vi "tracking+matching_gige_mit_5_pattern.vi"() -> ()   [LabVIEW 2014]
uses:
  <vilib>/userdefined/High Color/IMAQdx.ctl
  <vilib>/vision/Avi1.llb/AviRefnum.ctl
  <vilib>/vision/driver/NI_Vision_Acquisition_Software.lvlib
  <vilib>/vision/NI_Vision_Development_Module.lvlib
  <resource>/objmgr/imaqdx.rc
panel:
  in  "Max Data Size":u32=10000
  out "Selected Path":path
  in  "Frames Per Second":u32=20
  in  "BayerPattern":u32(ring)=5 items=["None", "GB", "GR", "BG", "RG", "Use Hardware Value"]
  out "ValueString":string
  out "ValueBool":bool
  out "IPAddress":string
  in  "Aufnahme Starten":bool
  in  "pattern5":bool
  in  "Pattern5 Farbe":u32(colorbox)=16711680
  in  "y":i32
  in  "x":i32
  out "Pattern 5":T1(plugin-control)
  in  "Template File Path (Pattern Matching 5)":path=path "C:/Users/Kroll/Desktop/Test_04012016/Pattern/pattern_1412.png"
  in  "pattern4":bool
  in  "Pattern4 Farbe":u32(colorbox)=16711680
  in  "y":i32
  in  "x":i32
  out "Pattern 4":T1(plugin-control)
  in  "Template File Path (Pattern Matching 4)":path=path "C:/Users/Kroll/Desktop/Test_04012016/Pattern/pattern_1412.png"
  in  "pattern3":bool
  in  "Pattern3 Farbe":u32(colorbox)=16711680
  in  "y":i32
  in  "x":i32
  out "Pattern 3":T1(plugin-control)
  in  "Template File Path (Pattern Matching 3)":path=path "C:/Users/Kroll/Desktop/Test_04012016/Pattern/pattern_1412.png"
  in  "pattern2":bool
  in  "Pattern2 Farbe":u32(colorbox)=16711680
  in  "x":i32
  in  "y":i32
  out "Pattern 2":T1(plugin-control)
  in  "Template File Path (Pattern Matching 2)":path=path "C:/Users/Kroll/Desktop/Test_04012016/Pattern/pattern_1412.png"
  out "date/time string":string
  in  "file path (dialog if empty)":path=path "I:/123.txt"
  in  "Länge der Spur":i32=50
  out "Pattern1":T1(plugin-control)
  in  "Template File Path (Pattern Matching 1)":path=path "C:/Users/Kroll/Desktop/Test_04012016/Pattern/pattern_1412.png"
  out "Image 2":T1(plugin-control)
  in  "Programm anhalten":bool
  in  "Parameters Pattern":T2={"Number of Matches Requested"=1, "Minimum Match Score"=800.0, "Angle Ranges"=[{"Start Angle"=-180.0, "End Angle"=180.0}, {"Start Angle"=0.0, "End Angle"=360.0}]}
  in  "Mittelpunktgröße":sgl
  in  "millisecond multiple":u32
  out "Processed Frames/s":dbl
  in  "Länge des Pfeils":sgl=80.0
  out "Acquired Frames/s":dbl
  in  "pattern1":bool
  in  "Pattern1 Farbe":u32(colorbox)=16711680
  in  "x":i32
  in  "y":i32
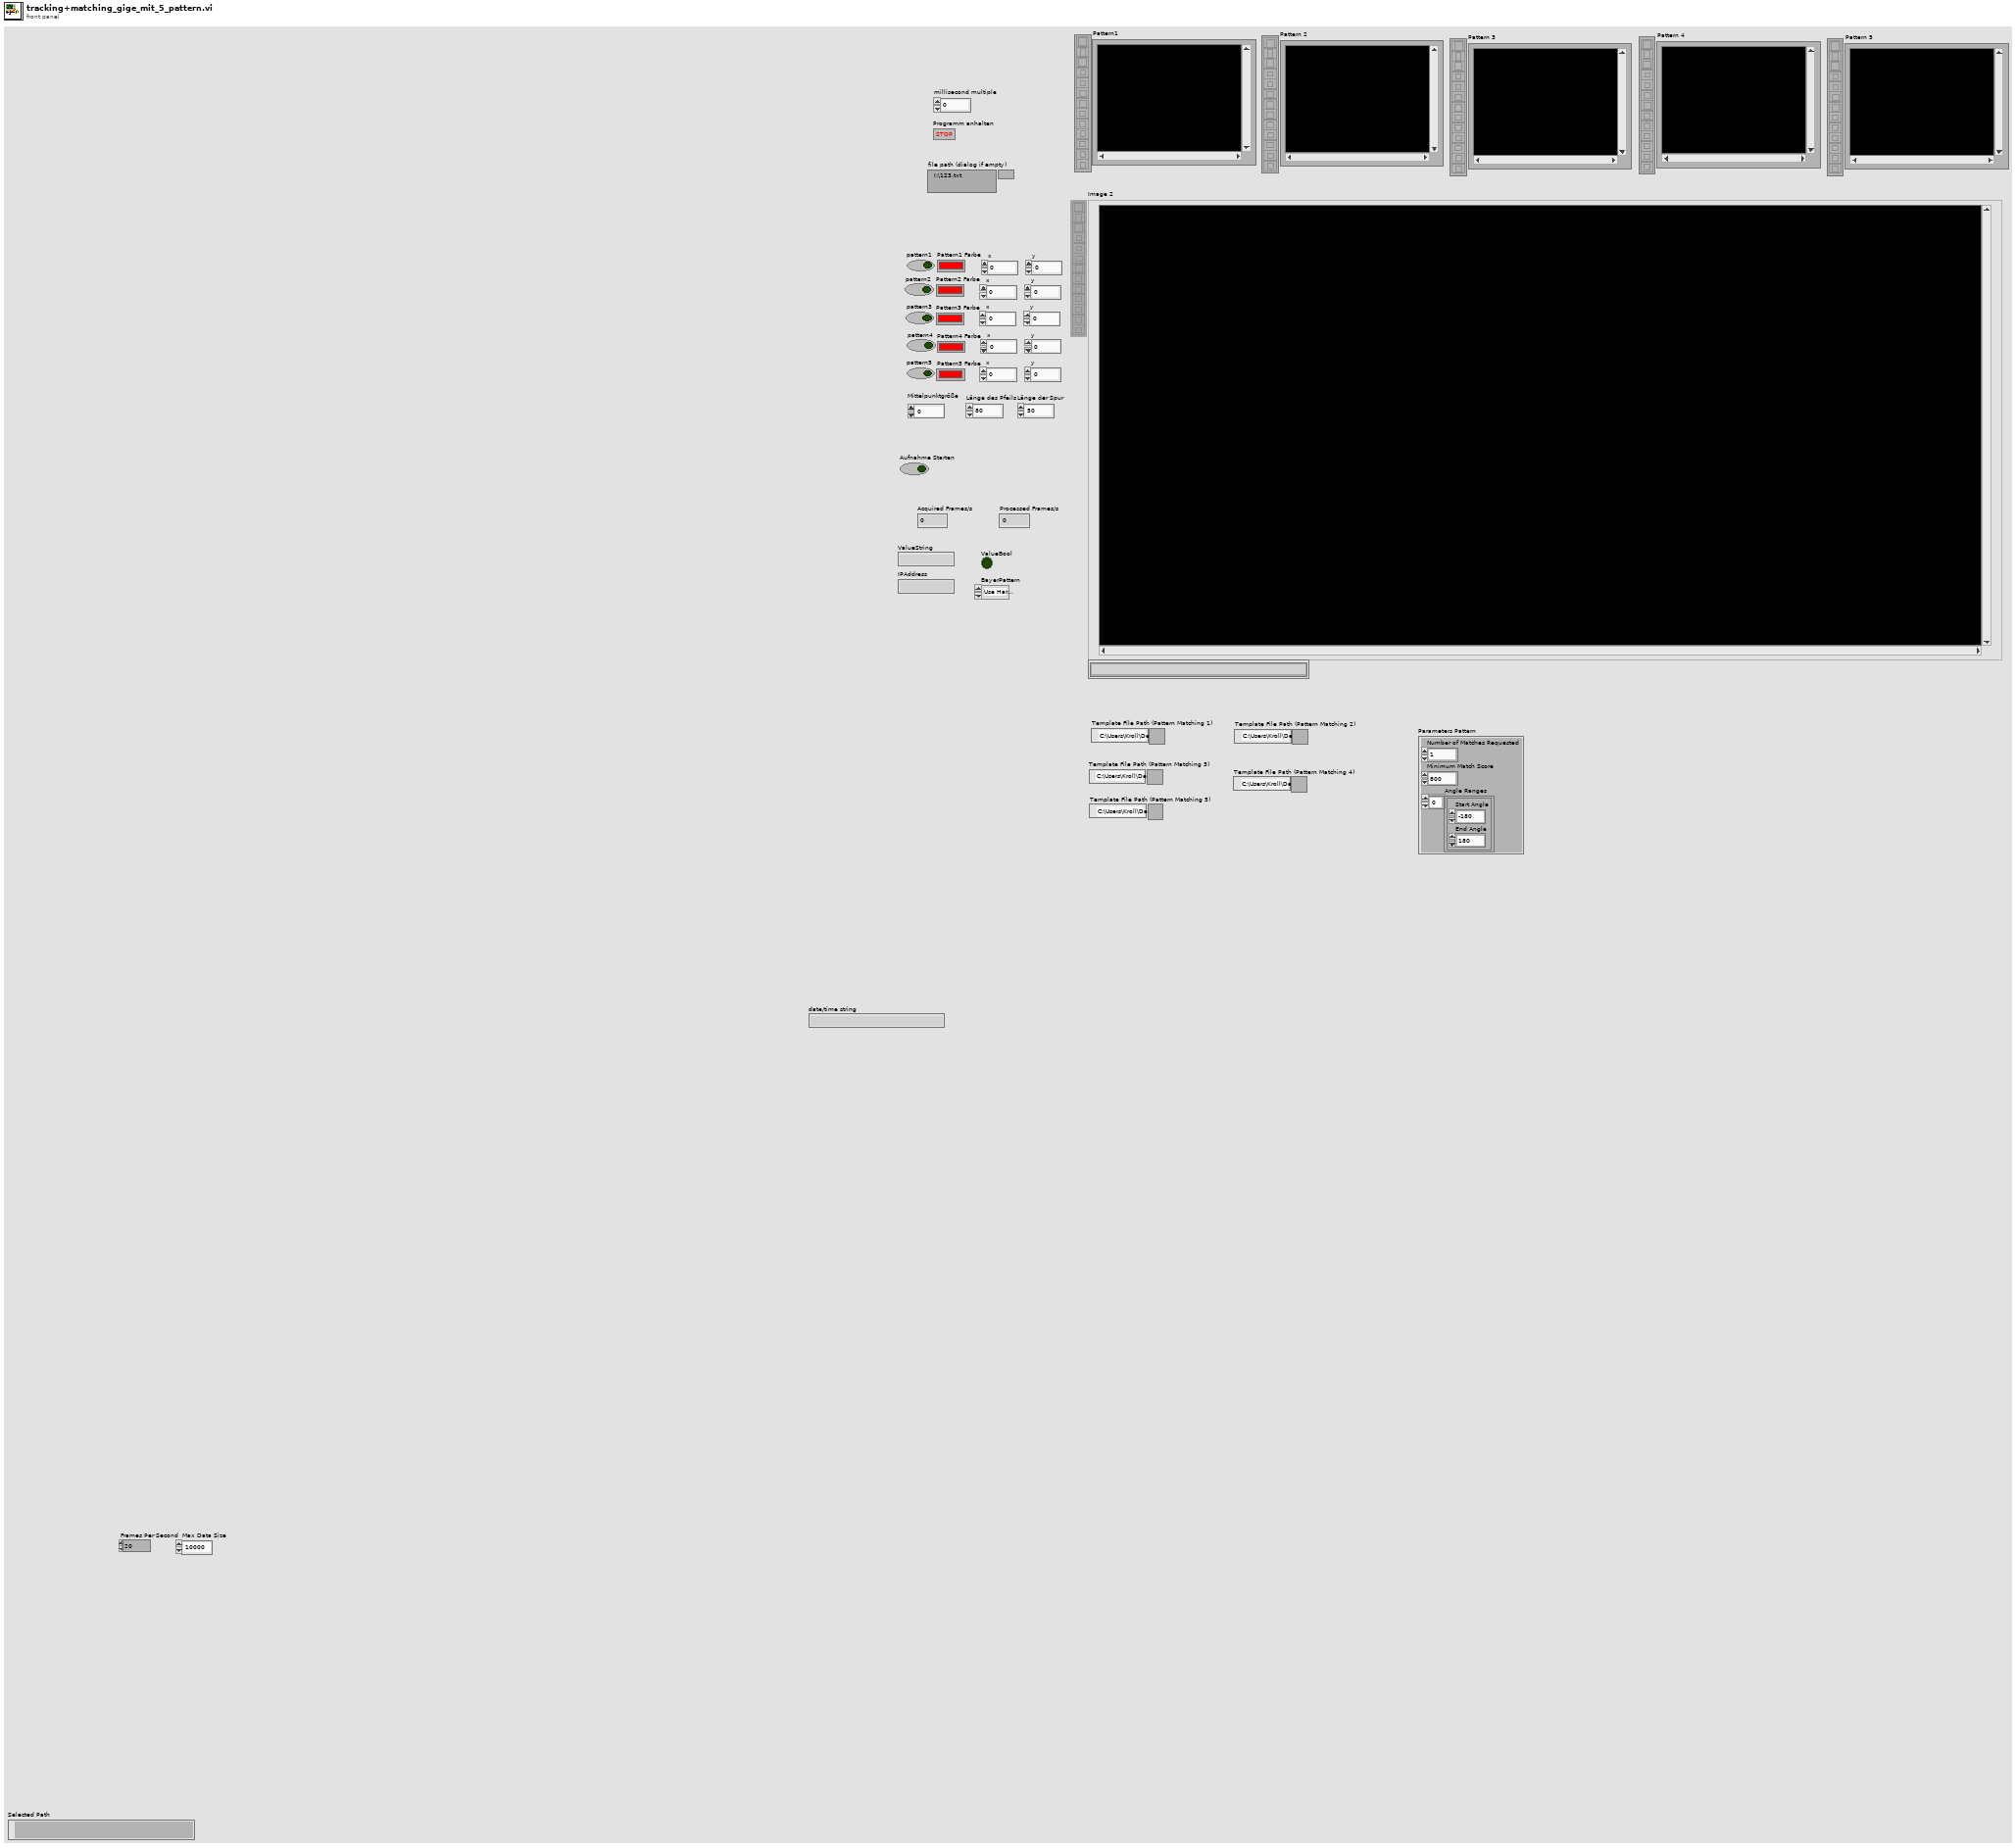
[diagram p1: front panel]
types:
  T1 = typedef "IMAQ Image.ctl" = refnum<image>
  T2 = cluster{"Number of Matches Requested":i32, "Minimum Match Score":sgl, "Angle Ranges":cluster{"Start Angle":sgl, "End Angle":sgl}[]}
  T3 = typedef "IMAQdx.ctl" = refnum<k21>
  T4 = cluster{"Number of Histogram Bins":i32, "Blending Parameter (%)":dbl, "Maximum Iterations":i32}
  T5 = typedef "Image Type" = u32
  T6 = enum16{"open", "replace", "create", "open or create", "replace or create", "replace or create with confirmation"}
  T7 = typedef "AviRefnum.ctl" = refnum<k1>
  T8 = enum32{"existing file", "new file", "new or existing file", "existing dir", "new dir", "new or existing dir", "existing file (use LLBs)", "new file (use LLBs)", "new or existing file (use LLBs)", "new or existing file or directory (use LLBs)"}
  T9 = typedef "IMAQ Object Tracking Session.ctl" = refnum<k20>
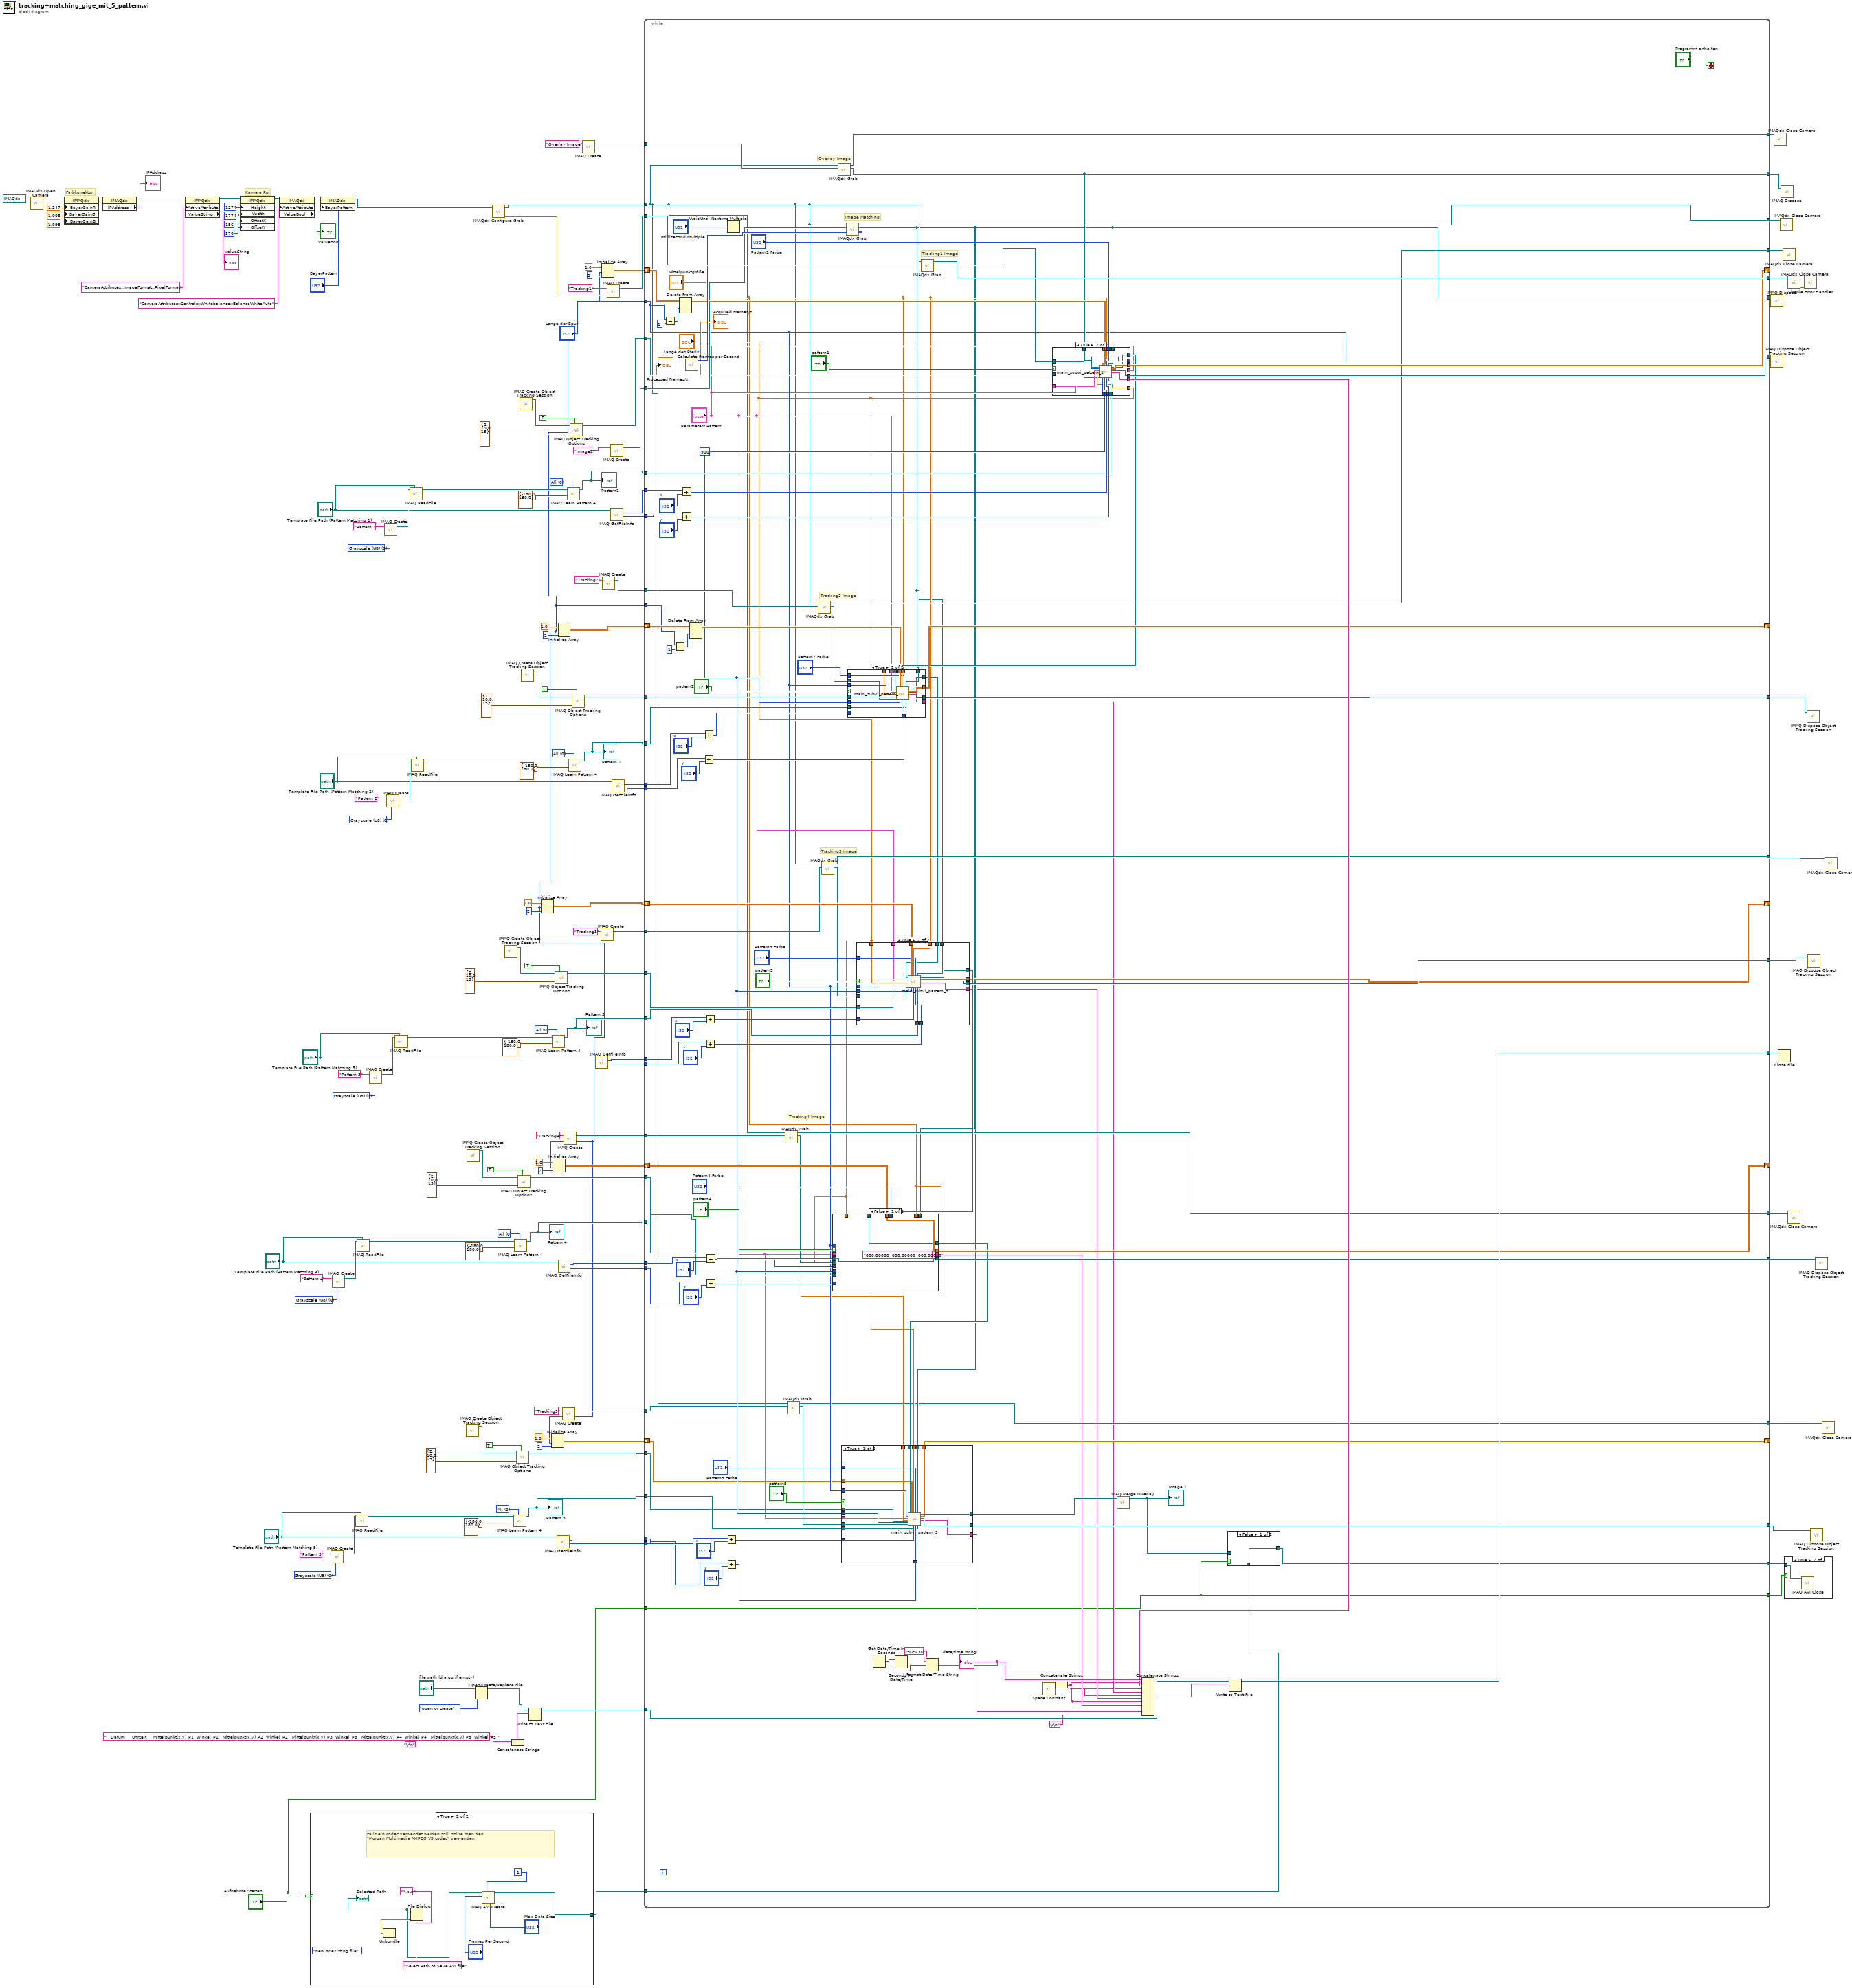
[diagram p0: block diagram]
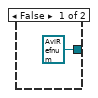
[diagram p2: hidden frame]
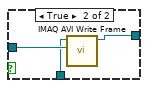
[diagram p4: hidden frame]
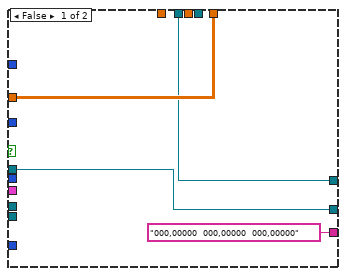
[diagram p5: hidden frame]
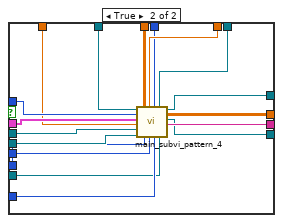
[diagram p6: hidden frame]
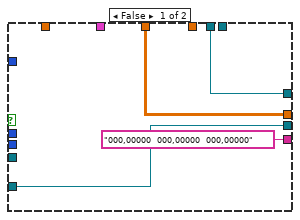
[diagram p7: hidden frame]
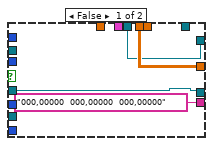
[diagram p8: hidden frame]
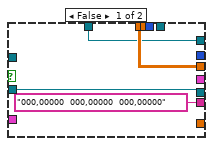
[diagram p9: hidden frame]
diagram:
  w43 = T5 0 items=["Grayscale (U8)", "Grayscale (I16)", "Grayscale (SGL)", "Complex (CSG)", "RGB (U32)", "HSL (U32)", "RGB (U64)", "Grayscale (U16)"] ("Image Type")
  w47 = 0 items=["All", "Low Discrepancy Sampling", "Grayscale Value Pyramid", "Gradients Pyramid"] ("Algorithm")
  w64 = T5 0 items=["Grayscale (U8)", "Grayscale (I16)", "Grayscale (SGL)", "Complex (CSG)", "RGB (U32)", "HSL (U32)", "RGB (U64)", "Grayscale (U16)"] ("Image Type")
  w68 = 0 items=["All", "Low Discrepancy Sampling", "Grayscale Value Pyramid", "Gradients Pyramid"] ("Algorithm")
  w88 = T5 0 items=["Grayscale (U8)", "Grayscale (I16)", "Grayscale (SGL)", "Complex (CSG)", "RGB (U32)", "HSL (U32)", "RGB (U64)", "Grayscale (U16)"] ("Image Type")
  w92 = 0 items=["All", "Low Discrepancy Sampling", "Grayscale Value Pyramid", "Gradients Pyramid"] ("Algorithm")
  w107 = T5 0 items=["Grayscale (U8)", "Grayscale (I16)", "Grayscale (SGL)", "Complex (CSG)", "RGB (U32)", "HSL (U32)", "RGB (U64)", "Grayscale (U16)"] ("Image Type")
  w111 = 0 items=["All", "Low Discrepancy Sampling", "Grayscale Value Pyramid", "Gradients Pyramid"] ("Algorithm")
  w132 = T5 0 items=["Grayscale (U8)", "Grayscale (I16)", "Grayscale (SGL)", "Complex (CSG)", "RGB (U32)", "HSL (U32)", "RGB (U64)", "Grayscale (U16)"] ("Image Type")
  w136 = 0 items=["All", "Low Discrepancy Sampling", "Grayscale Value Pyramid", "Gradients Pyramid"] ("Algorithm")
  # "Kamera Roi"
  # "Farbkorrektur"
  n1 = call <vilib>:"IMAQdx Open Camera.vi"("Session In"=T3 "cam0") -> ("Session Out"=w13:T3)  [unwired: 9 in, 1 out]
  n2 = property class="IMAQdx"(reference=w13, "BayerGainR"=1.247, "BayerGainG"=1.003, "BayerGainB"=1.098) -> (reference out=w17:T3)  [unwired: 1 in, 1 out]
  n3 = property class="IMAQdx"(reference=w17) -> (reference out=w5:T3, "IPAddress"=→"IPAddress":string)  [unwired: 1 in, 1 out]
  n4 = property class="IMAQdx"(reference=w5, "ActiveAttribute"="CameraAttributes::ImageFormat::PixelFormat") -> (reference out=w10:T3, "ValueString"=→"ValueString":string)  [unwired: 1 in, 1 out]
  n5 = property class="IMAQdx"(reference=w10, "Height"=u32 1274, "Width"=u32 1774, "OffsetX"=u32 156, "OffsetY"=u32 370) -> (reference out=w11:T3)  [unwired: 1 in, 1 out]
  n6 = property class="IMAQdx"(reference=w11, "ActiveAttribute"="CameraAttributes::Controls::Whitebalance::BalanceWhiteAuto") -> (reference out=w21:T3, "ValueBool"=→"ValueBool":bool)  [unwired: 1 in, 1 out]
  n7 = case shown="True" "Aufnahme Starten" {
    tunnel: [T7 refnum ("Avi Refnum") w153] -> w3
    frame False {
    }
    frame True {
      (unwired) T8."new or existing file" ("select mode (2)")
      # "Falls ein codec verwendet werden soll, sollte man den \n\"Morgan Multimedia M-JPEG V3 codec\" verwenden"
      n8 = File Dialog(6:"*.avi" ("pattern"), 7:"Select Path to Save AVI file" ("prompt")) -> (0:w156:errorcluster, 3:w155:path)  [unwired: 1 in, 6 out]
      "Selected Path" <- w155
      n9 = Unbundle(w156) -> ()  [unwired: 3 out]
      n10 = call "IMAQ AVI Create"("Max Data Size"="Max Data Size", "quality"=-1, "Frames Per Second"="Frames Per Second", "AVI Path"=w155) -> ("Avi Refnum"=w153:T7)  [unwired: 6 in, 1 out]
    }
  }
  n11 = property class="IMAQdx"(reference=w21, "BayerPattern"="BayerPattern") -> (reference out=w4:T3)  [unwired: 1 in, 1 out]
  n12 = call "IMAQ Create"("Image Name"="Pattern 5", "Image Type"=w43) -> ("New Image"=w44:T1)  [unwired: 3 in, 1 out]
  n13 = call "IMAQ Create"("Image Name"="Pattern 4", "Image Type"=w64) -> ("New Image"=w65:T1)  [unwired: 3 in, 1 out]
  n14 = call "IMAQ ReadFile"("File Path"="Template File Path (Pattern Matching 5)", "Image"=w44) -> ("Image Out"=w41:T1)  [unwired: 5 in, 4 out]
  n15 = call "IMAQ ReadFile"("File Path"="Template File Path (Pattern Matching 4)", "Image"=w65) -> ("Image Out"=w62:T1)  [unwired: 5 in, 4 out]
  n16 = call "IMAQ Create"("Image Name"="Pattern 3", "Image Type"=w88) -> ("New Image"=w89:T1)  [unwired: 3 in, 1 out]
  n17 = call "IMAQ Create"("Image Name"="Pattern 1", "Image Type"=w132) -> ("New Image"=w133:T1)  [unwired: 3 in, 1 out]
  n18 = call "IMAQ Create"("Image Name"="Pattern 2", "Image Type"=w107) -> ("New Image"=w108:T1)  [unwired: 3 in, 1 out]
  n19 = call "IMAQ ReadFile"("File Path"="Template File Path (Pattern Matching 3)", "Image"=w89) -> ("Image Out"=w86:T1)  [unwired: 5 in, 4 out]
  n20 = call "IMAQ ReadFile"("File Path"="Template File Path (Pattern Matching 1)", "Image"=w133) -> ("Image Out"=w129:T1)  [unwired: 5 in, 4 out]
  n21 = call "IMAQ ReadFile"("File Path"="Template File Path (Pattern Matching 2)", "Image"=w108) -> ("Image Out"=w105:T1)  [unwired: 5 in, 4 out]
  n22 = call "IMAQ Create Object Tracking Session"() -> ("Object Tracking Session"=w40:T9)  [unwired: 1 in, 10 out]
  n23 = call "IMAQ Create Object Tracking Session"() -> ("Object Tracking Session"=w61:T9)  [unwired: 1 in, 10 out]
  n24 = Open/Create/Replace File(file path (use dialog)="file path (dialog if empty)", operation (0:open)=T6."open or create") -> (refnum out=w118:refnum<file>)  [unwired: 4 in, 2 out]
  n25 = call <vilib>:"IMAQdx Configure Grab.vi"("Session In"=w4) -> ("error out"=w150:errorcluster, "Session Out"=w148:T3)  [unwired: 9 in]
  n26 = call "IMAQ Create Object Tracking Session"() -> ("Object Tracking Session"=w85:T9)  [unwired: 1 in, 10 out]
  n27 = Concatenate Strings("   Datum     Uhrzeit     Mittelpunkt(x,y)_P1  Winkel_P1   Mittelpunkt(x,y)_P2  Winkel_P2   Mittelpunkt(x,y)_P3  Winkel_P3   Mittelpunkt(x,y)_P4  Winkel_P4   Mittelpunkt(x,y)_P5  Winkel_P5 " ("string"), "\r\n") -> (w116:string)
  n28 = call "IMAQ Learn Pattern 4"("Algorithm"=w47, "Angle Range"=cluster{"Start Angle":sgl, "End Angle":sgl} {"Start Angle"=-180.0, "End Angle"=180.0}, "Image"=w41) -> ("Template Image Out"=w31:T1)  [unwired: 6 in, 2 out]
  "Pattern 5" <- w31
  n29 = call "IMAQ Learn Pattern 4"("Algorithm"=w68, "Angle Range"=cluster{"Start Angle":sgl, "End Angle":sgl} {"Start Angle"=-180.0, "End Angle"=180.0}, "Image"=w62) -> ("Template Image Out"=w55:T1)  [unwired: 6 in, 2 out]
  "Pattern 4" <- w55
  n30 = call-poly "IMAQ Object Tracking Options"("Get/Set (Get)"=TRUE, "Mean Shift Options in"=T4 {"Number of Histogram Bins"=2, "Blending Parameter (%)"=10.0, "Maximum Iterations"=15}, "Object Tracking Session In"=w40) -> ("Object Tracking Session Out"=w32:T9)  [unwired: 6 in, 2 out]
  n31 = call-poly "IMAQ Object Tracking Options"("Get/Set (Get)"=TRUE, "Mean Shift Options in"=T4 {"Number of Histogram Bins"=2, "Blending Parameter (%)"=10.0, "Maximum Iterations"=15}, "Object Tracking Session In"=w61) -> ("Object Tracking Session Out"=w56:T9)  [unwired: 6 in, 2 out]
  n32 = call "IMAQ Create Object Tracking Session"() -> ("Object Tracking Session"=w128:T9)  [unwired: 1 in, 10 out]
  n33 = call "IMAQ Create Object Tracking Session"() -> ("Object Tracking Session"=w104:T9)  [unwired: 1 in, 10 out]
  n34 = Write to Text File(file (use dialog)=w118, text=w116) -> (refnum out=w114:refnum<file>)  [unwired: 2 in, 2 out]
  n35 = Initialize Array "Initialize Array"(1.0 ("element"), "Länge der Spur", 2 ("dimension size")) -> (w80:dbl[][])
  n36 = Initialize Array "Initialize Array"(1.0 ("element"), "Länge der Spur", 2 ("dimension size")) -> (w33:dbl[][])
  n37 = call "IMAQ Learn Pattern 4"("Algorithm"=w92, "Angle Range"=cluster{"Start Angle":sgl, "End Angle":sgl} {"Start Angle"=-180.0, "End Angle"=180.0}, "Image"=w86) -> ("Template Image Out"=w78:T1)  [unwired: 6 in, 2 out]
  "Pattern 3" <- w78
  n38 = Initialize Array "Initialize Array"(1.0 ("element"), "Länge der Spur", 2 ("dimension size")) -> (w50:dbl[][])
  n39 = call-poly "IMAQ Object Tracking Options"("Get/Set (Get)"=TRUE, "Mean Shift Options in"=T4 {"Number of Histogram Bins"=2, "Blending Parameter (%)"=10.0, "Maximum Iterations"=15}, "Object Tracking Session In"=w85) -> ("Object Tracking Session Out"=w79:T9)  [unwired: 6 in, 2 out]
  n40 = call "IMAQ GetFileInfo"("File Path"="Template File Path (Pattern Matching 5)") -> ("Y Resolution"=w29:i32, "X Resolution"=w30:i32)  [unwired: 4 in, 5 out]
  n41 = Initialize Array "Initialize Array"(1.0 ("element"), "Länge der Spur", 2 ("dimension size")) -> (w95:dbl[][])
  n42 = call "IMAQ GetFileInfo"("File Path"="Template File Path (Pattern Matching 4)") -> ("Y Resolution"=w53:i32, "X Resolution"=w54:i32)  [unwired: 4 in, 5 out]
  n43 = call "IMAQ Create"("Image Name"="Tracking5") -> ("New Image"=w34:T1)  [unwired: 4 in, 1 out]
  n44 = call "IMAQ Create"("Image Name"="Tracking4") -> ("New Image"=w57:T1)  [unwired: 4 in, 1 out]
  n45 = call "IMAQ Learn Pattern 4"("Algorithm"=w136, "Angle Range"=cluster{"Start Angle":sgl, "End Angle":sgl} {"Start Angle"=-180.0, "End Angle"=180.0}, "Image"=w129) -> ("Template Image Out"=w130:T1)  [unwired: 6 in, 2 out]
  "Pattern1" <- w130
  n46 = call "IMAQ Learn Pattern 4"("Algorithm"=w111, "Angle Range"=cluster{"Start Angle":sgl, "End Angle":sgl} {"Start Angle"=-180.0, "End Angle"=180.0}, "Image"=w105) -> ("Template Image Out"=w100:T1)  [unwired: 6 in, 2 out]
  "Pattern 2" <- w100
  n47 = call-poly "IMAQ Object Tracking Options"("Get/Set (Get)"=TRUE, "Mean Shift Options in"=T4 {"Number of Histogram Bins"=2, "Blending Parameter (%)"=10.0, "Maximum Iterations"=15}, "Object Tracking Session In"=w128) -> ("Object Tracking Session Out"=w127:T9)  [unwired: 6 in, 2 out]
  n48 = call-poly "IMAQ Object Tracking Options"("Get/Set (Get)"=TRUE, "Mean Shift Options in"=T4 {"Number of Histogram Bins"=2, "Blending Parameter (%)"=10.0, "Maximum Iterations"=15}, "Object Tracking Session In"=w104) -> ("Object Tracking Session Out"=w101:T9)  [unwired: 6 in, 2 out]
  n49 = call "IMAQ Create"("Image Name"="Overlay Image") -> ("New Image"=w124:T1)  [unwired: 4 in, 1 out]
  n50 = call "IMAQ GetFileInfo"("File Path"="Template File Path (Pattern Matching 3)") -> ("Y Resolution"=w76:i32, "X Resolution"=w77:i32)  [unwired: 4 in, 5 out]
  n51 = call "IMAQ Create"("Image Name"="Tracking3") -> ("New Image"=w70:T1)  [unwired: 4 in, 1 out]
  n52 = Initialize Array "Initialize Array"(1.0 ("element"), "Länge der Spur", 2 ("dimension size")) -> (w138:dbl[][])
  n53 = call "IMAQ Create"("Image Name"="Tracking2") -> ("New Image"=w93:T1)  [unwired: 4 in, 1 out]
  n54 = call "IMAQ Create"("Image Name"="Tracking1", "error in (no error)"=w150) -> ("New Image"=w147:T1)  [unwired: 3 in, 1 out]
  n55 = call "IMAQ Create"("Image Name"="image2") -> ("New Image"=w143:T1)  [unwired: 4 in, 1 out]
  n56 = call "IMAQ GetFileInfo"("File Path"="Template File Path (Pattern Matching 1)") -> ("Y Resolution"=w140:i32, "X Resolution"=w141:i32)  [unwired: 4 in, 5 out]
  n57 = call "IMAQ GetFileInfo"("File Path"="Template File Path (Pattern Matching 2)") -> ("Y Resolution"=w98:i32, "X Resolution"=w99:i32)  [unwired: 4 in, 5 out]
  n58 = while {
    tunnel: w148 -> [w178]
    tunnel: w147 -> [w285]
    tunnel: [w286] -> w145
    tunnel: [w174] -> w142
    tunnel: w143 -> [w271]
    tunnel: w141 -> [w272]
    tunnel: w140 -> [w273]
    shift-right: [w264] -> _
    shift-left: w138 -> [w280]
    tunnel: "Länge der Spur" -> [w187]
    tunnel: w130 -> [w261]
    tunnel: w127 -> [w265]
    tunnel: [w270] -> w125
    tunnel: w124 -> [w267]
    tunnel: [w262] -> w123
    tunnel: [w266] -> w122
    tunnel: w114 -> [w258]
    tunnel: [w254] -> w113
    tunnel: w101 -> [w242]
    tunnel: w100 -> [w239]
    tunnel: w99 -> [w251]
    tunnel: w98 -> [w250]
    shift-right: [w244] -> _
    shift-left: w95 -> [w247]
    tunnel: "Länge der Spur" -> [w246]
    tunnel: w93 -> [w234]
    tunnel: w79 -> [w221]
    tunnel: w78 -> [w225]
    tunnel: w77 -> [w231]
    tunnel: w76 -> [w230]
    tunnel: [w220] -> w75
    tunnel: [w219] -> w74
    tunnel: [w218] -> w73
    tunnel: [w217] -> w72
    tunnel: w70 -> [w216]
    tunnel: [w214] -> w69
    tunnel: w57 -> [w209]
    tunnel: w56 -> [w204]
    tunnel: w55 -> [w200]
    tunnel: w54 -> [w211]
    tunnel: w53 -> [w210]
    tunnel: [w199] -> w49
    tunnel: [w198] -> w48
    shift-right: [w196] -> _
    shift-left: w80 -> [w229]
    shift-right: [w195] -> _
    shift-left: w50 -> [w208]
    tunnel: w34 -> [w177]
    shift-right: [w181] -> _
    shift-left: w33 -> [w182]
    tunnel: w32 -> [w172]
    tunnel: w31 -> [w175]
    tunnel: w30 -> [w192]
    tunnel: w29 -> [w191]
    tunnel: [w173] -> w27
    tunnel: [w171] -> w26
    tunnel: w3 -> [w160]
    tunnel: "Aufnahme Starten" -> [w162]
    tunnel: [w162] -> w25
    tunnel: [w163] -> w1
    stop <- "Programm anhalten" stop-if-true
    w188 = 900 ("Minimum Score")
    # "Tracking4 Image"
    # "Tracking3 Image"
    # "Tracking2 Image"
    # "Overlay Image"
    # "Image Matching"
    # "Tracking1 Image"
    n59 = Subtract(x=w187, y=1) -> (x-y=w277:i32)
    n60 = Subtract(x=w246, y=1) -> (x-y=w248:i32)
    n61 = Delete From Array "Delete From Array"(array=w280, index (row)=w277) -> (array with subset deleted=w279:dbl[][])  [unwired: 2 in, 1 out]
    n62 = Add(x=w272, y="x") -> (x+y=w269:i32)
    n63 = Add(x=w273, y="y") -> (x+y=w268:i32)
    n64 = Delete From Array "Delete From Array"(array=w247, index (row)=w248) -> (array with subset deleted=w245:dbl[][])  [unwired: 2 in, 1 out]
    n65 = Add(x=w251, y="x") -> (x+y=w240:i32)
    n66 = Add(x=w250, y="y") -> (x+y=w241:i32)
    n67 = Add(x=w231, y="x") -> (x+y=w224:i32)
    n68 = Add(x=w230, y="y") -> (x+y=w223:i32)
    n69 = Add(x=w211, y="x") -> (x+y=w202:i32)
    n70 = Add(x=w210, y="y") -> (x+y=w201:i32)
    n71 = Add(x=w192, y="x") -> (x+y=w189:i32)
    n72 = Add(x=w191, y="y") -> (x+y=w190:i32)
    n73 = Wait Until Next ms Multiple(millisecond multiple="millisecond multiple") -> ()  [unwired: 1 out]
    n74 = call <vilib>:"IMAQdx Grab.vi"("Image In"=w209, "Session In"=w178) -> ("Image Out"=w203:T1, "Session Out"=w198:T3)  [unwired: 6 in, 2 out]
    n75 = call <vilib>:"IMAQdx Grab.vi"("Image In"=w177, "Session In"=w178) -> ("Image Out"=w176:T1, "Session Out"=w171:T3)  [unwired: 6 in, 2 out]
    n76 = call <vilib>:"IMAQdx Grab.vi"("Image In"=w234, "Session In"=w178) -> ("Image Out"=w222:T1, "Session Out"=w218:T3)  [unwired: 6 in, 2 out]
    n77 = call <vilib>:"IMAQdx Grab.vi"("Image In"=w216, "Session In"=w178) -> ("Image Out"=w215:T1, "Session Out"=w214:T3)  [unwired: 6 in, 2 out]
    n78 = call <vilib>:"IMAQdx Grab.vi"("Image In"=w267, "Session In"=w178) -> ("Image Out"=w262:T1, "Session Out"=w266:T3)  [unwired: 6 in, 2 out]
    n79 = call <vilib>:"IMAQdx Grab.vi"("Image In"=w271, "Session In"=w178) -> ("Buffer Number Out"=w283:u32, "Image Out"=w174:T1, "Session Out"=w217:T3)  [unwired: 6 in, 1 out]
    n80 = call <vilib>:"Calculate Frames per Second.vi"("Buffer Number"=w283) -> ("Processed Frames/s"=→"Processed Frames/s":dbl, "Acquired Frames/s"=→"Acquired Frames/s":dbl)  [unwired: 8 in, 1 out]
    n81 = Get Date/Time In Seconds() -> (seconds since 1Jan1904=w257:timestamp)
    n82 = Seconds To Date/Time(time stamp (now)=w257) -> ()  [unwired: 1 in, 1 out]
    n83 = call <vilib>:"IMAQdx Grab.vi"("Image In"=w285, "Session In"=w178) -> ("Image Out"=w238:T1, "Session Out"=w286:T3)  [unwired: 6 in, 2 out]
    n84 = Format Date/Time String(time format string (%c)="%c%3u", seconds (now)=w257) -> (date/time string=w255:string)  [unwired: 1 in]
    "date/time string" <- w255
    n85 = call <vilib>:"Space Constant.vi"() -> ("String"=w260:string)
    n86 = case shown="True" "pattern1" {
      tunnel: w279 -> [w381 w392]
      tunnel: "Länge des Pfeils" -> [_ w388]
      tunnel: "Mittelpunktgröße" -> [_ w391]
      tunnel: w188 -> [_ w394]
      tunnel: [w382 w399] -> w270
      tunnel: w269 -> [_ w395]
      tunnel: w268 -> [_ w396]
      tunnel: w265 -> [w382 w393]
      tunnel: w187 -> [_ w385]
      tunnel: [w381 w400] -> w264
      tunnel: "Pattern1 Farbe" -> [_ w386]
      tunnel: w262 -> [w379 w390]
      tunnel: w261 -> [_ w397]
      tunnel: ["000,00000  000,00000  000,00000" ("String") w398] -> w253
      tunnel: "Parameters Pattern" -> [_ _]
      tunnel: [w379 w384] -> w226
      tunnel: w238 -> [_ w387]
      tunnel: "Parameters Pattern" -> [_ w389]
      tunnel: w174 -> [_ w383]
      frame False {
      }
      frame True {
        n87 = call "main_subvi_pattern_1.vi"("Refnum Original Bild"=w390, "Länge der Spur"=w385, "Parameters Pattern"=w389, "Länge des Pfeils"=w388, "Object Tracking Session Out in"=w393, "Refnum Tracking"=w387, "Array in"=w392, "Minimum Score"=w394, "Mittelpunktgröße"=w391, "Numeric 2"=w395, "Pattern1 Farbe"=w386, "Numeric"=w396, "Image Matching"=w383, "Template Image In"=w397) -> ("Refnum OUt"=w384:T1, "Array out"=w400:dbl[][], "Object Tracking Session Out out"=w399:T9, "String"=w398:string)  [unwired: 2 in]
      }
    }
    n88 = case shown="True" "pattern2" {
      tunnel: [w358 w378] -> w220
      tunnel: [w359 w377] -> w244
      tunnel: ["000,00000  000,00000  000,00000" ("String") w376] -> w169
      tunnel: [w357 w375] -> w197
      tunnel: w245 -> [w359 w374]
      tunnel: w174 -> [_ w373]
      tunnel: "Mittelpunktgröße" -> [_ w372]
      tunnel: "Pattern2 Farbe" -> [_ w371]
      tunnel: w187 -> [_ w370]
      tunnel: w242 -> [w358 w369]
      tunnel: w226 -> [w357 w368]
      tunnel: "Parameters Pattern" -> [_ w367]
      tunnel: w188 -> [_ w366]
      tunnel: w241 -> [_ w365]
      tunnel: w240 -> [_ w364]
      tunnel: w239 -> [_ w363]
      tunnel: "Länge des Pfeils" -> [_ w362]
      tunnel: w222 -> [_ w361]
      frame False {
      }
      frame True {
        n89 = call "main_subvi_pattern_2.vi"("Refnum Original Bild"=w368, "Länge der Spur"=w370, "Parameters Pattern"=w367, "Länge des Pfeils"=w362, "Object Tracking Session Out in"=w369, "Refnum Tracking"=w361, "Array in"=w374, "Minimum Score"=w366, "Mittelpunktgröße"=w372, "Numeric 2"=w364, "Pattern1 Farbe"=w371, "Numeric"=w365, "Image Matching"=w373, "Template Image In"=w363) -> ("Refnum OUt"=w375:T1, "Array out"=w377:dbl[][], "Object Tracking Session Out out"=w378:T9, "String"=w376:string)  [unwired: 2 in]
      }
    }
    n90 = case shown="True" "pattern3" {
      tunnel: w229 -> [w336 w356]
      tunnel: "Mittelpunktgröße" -> [_ w355]
      tunnel: "Pattern3 Farbe" -> [_ w354]
      tunnel: [w335 w353] -> w206
      tunnel: [w336 w352] -> w196
      tunnel: w187 -> [_ w351]
      tunnel: [w337 w350] -> w219
      tunnel: ["000,00000  000,00000  000,00000" ("String") w349] -> w168
      tunnel: w225 -> [_ w348]
      tunnel: w224 -> [_ w347]
      tunnel: w223 -> [_ w346]
      tunnel: w188 -> [_ w345]
      tunnel: w215 -> [_ w344]
      tunnel: w221 -> [w337 w343]
      tunnel: "Parameters Pattern" -> [_ w342]
      tunnel: "Länge des Pfeils" -> [_ w341]
      tunnel: w174 -> [_ w340]
      tunnel: w197 -> [w335 w339]
      frame False {
      }
      frame True {
        n91 = call "main_subvi_pattern_3.vi"("Refnum Original Bild"=w339, "Länge der Spur"=w351, "Parameters Pattern"=w342, "Länge des Pfeils"=w341, "Object Tracking Session Out in"=w343, "Refnum Tracking"=w344, "Array in"=w356, "Minimum Score"=w345, "Mittelpunktgröße"=w355, "Numeric 2"=w347, "Pattern1 Farbe"=w354, "Numeric"=w346, "Image Matching"=w340, "Template Image In"=w348) -> ("Refnum OUt"=w353:T1, "Array out"=w352:dbl[][], "Object Tracking Session Out out"=w350:T9, "String"=w349:string)  [unwired: 2 in]
      }
    }
    n92 = case shown="False" "pattern4" {
      tunnel: w208 -> [w314 w334]
      tunnel: "Mittelpunktgröße" -> [_ w333]
      tunnel: "Pattern4 Farbe" -> [_ w332]
      tunnel: w206 -> [w313 w331]
      tunnel: [w314 w330] -> w195
      tunnel: w187 -> [_ w329]
      tunnel: "Parameters Pattern" -> [_ w328]
      tunnel: "Länge des Pfeils" -> [_ w327]
      tunnel: w204 -> [w315 w326]
      tunnel: w203 -> [_ w325]
      tunnel: w188 -> [_ w324]
      tunnel: w202 -> [_ w323]
      tunnel: w201 -> [_ w322]
      tunnel: w200 -> [_ w321]
      tunnel: ["000,00000  000,00000  000,00000" ("String") w320] -> w167
      tunnel: [w315 w319] -> w199
      tunnel: [w313 w318] -> w185
      tunnel: w174 -> [_ w317]
      frame False {
      }
      frame True {
        n93 = call "main_subvi_pattern_4.vi"("Refnum Original Bild"=w331, "Länge der Spur"=w329, "Parameters Pattern"=w328, "Länge des Pfeils"=w327, "Object Tracking Session Out in"=w326, "Refnum Tracking"=w325, "Array in"=w334, "Minimum Score"=w324, "Mittelpunktgröße"=w333, "Numeric 2"=w323, "Pattern1 Farbe"=w332, "Numeric"=w322, "Image Matching"=w317, "Template Image In"=w321) -> ("Refnum OUt"=w318:T1, "Array out"=w330:dbl[][], "Object Tracking Session Out out"=w319:T9, "String"=w320:string)  [unwired: 2 in]
      }
    }
    n94 = case shown="True" "pattern5" {
      tunnel: w190 -> [_ w312]
      tunnel: w189 -> [_ w311]
      tunnel: w188 -> [_ w310]
      tunnel: w187 -> [_ w309]
      tunnel: w185 -> [w293 w308]
      tunnel: [w293 w307] -> w170
      tunnel: "Parameters Pattern" -> [_ w306]
      tunnel: "Länge des Pfeils" -> [_ w305]
      tunnel: w182 -> [w294 w304]
      tunnel: [w294 w303] -> w181
      tunnel: "Mittelpunktgröße" -> [_ w302]
      tunnel: "Pattern5 Farbe" -> [_ w301]
      tunnel: w176 -> [_ w300]
      tunnel: w175 -> [_ w299]
      tunnel: w174 -> [_ w298]
      tunnel: [w292 w297] -> w173
      tunnel: ["000,00000  000,00000  000,00000" ("String") w296] -> w165
      tunnel: w172 -> [w292 w295]
      frame False {
      }
      frame True {
        n95 = call "main_subvi_pattern_5.vi"("Refnum Original Bild"=w308, "Länge der Spur"=w309, "Parameters Pattern"=w306, "Länge des Pfeils"=w305, "Object Tracking Session Out in"=w295, "Refnum Tracking"=w300, "Array in"=w304, "Minimum Score"=w310, "Mittelpunktgröße"=w302, "Numeric 2"=w311, "Pattern1 Farbe"=w301, "Numeric"=w312, "Image Matching"=w298, "Template Image In"=w299) -> ("Refnum OUt"=w307:T1, "Array out"=w303:dbl[][], "Object Tracking Session Out out"=w297:T9, "String"=w296:string)  [unwired: 2 in]
      }
    }
    n96 = Concatenate Strings(w260, w260) -> (w166:string)
    n97 = call "IMAQ Merge Overlay"("Image Src"=w170) -> ("Image Dst Out"=w161:T1)  [unwired: 9 in, 1 out]
    "Image 2" <- w161
    n98 = Concatenate Strings(w255, w166, w253, w166, w169, w166, w168, w166, w167, w166, w165, "\r\n") -> (w259:string)
    n99 = case shown="False" w162 {
      tunnel: [w287 w288] -> w163
      tunnel: w161 -> [_ w290]
      tunnel: w160 -> [w287 w289]
      frame False {
      }
      frame True {
        n100 = call "IMAQ AVI Write Frame"("Image"=w290, "Avi Refnum"=w289) -> ("Avi Refnum (duplicate)"=w288:T7)  [unwired: 8 in, 1 out]
      }
    }
    n101 = Write to Text File(file (use dialog)=w258, text=w259) -> (refnum out=w254:refnum<file>)  [unwired: 2 in, 2 out]
  }
  n102 = call "IMAQ Dispose"("Image"=w142) -> ()  [unwired: 5 in, 1 out]
  n103 = call "IMAQ Dispose Object Tracking Session"("Object Tracking Session"=w125) -> ()  [unwired: 1 in, 10 out]
  n104 = call <vilib>:"IMAQdx Close Camera.vi"("Session In"=w122) -> ()  [unwired: 10 in, 1 out]
  n105 = Close File(refnum=w113) -> ()  [unwired: 1 in, 2 out]
  n106 = call <vilib>:"IMAQdx Close Camera.vi"("Session In"=w72) -> ()  [unwired: 10 in, 1 out]
  n107 = call "IMAQ Dispose"("Image"=w123) -> ()  [unwired: 5 in, 1 out]
  n108 = call <vilib>:"IMAQdx Close Camera.vi"("Session In"=w73) -> ()  [unwired: 10 in, 1 out]
  n109 = case shown="True" w25 {
    tunnel: w1 -> [_ w401]
    frame False {
    }
    frame True {
      n110 = call "IMAQ AVI Close"("Avi Refnum"=w401) -> ()  [unwired: 10 in, 1 out]
    }
  }
  n111 = call <vilib>:"IMAQdx Close Camera.vi"("Session In"=w145) -> ("error out"=w146:errorcluster)  [unwired: 10 in]
  n112 = call <vilib>:"IMAQdx Close Camera.vi"("Session In"=w48) -> ()  [unwired: 10 in, 1 out]
  n113 = call <vilib>:"Simple Error Handler.vi"("error in (no error)"=w146) -> ()  [unwired: 4 in, 5 out]
  n114 = call "IMAQ Dispose Object Tracking Session"("Object Tracking Session"=w75) -> ()  [unwired: 1 in, 10 out]
  n115 = call "IMAQ Dispose Object Tracking Session"("Object Tracking Session"=w74) -> ()  [unwired: 1 in, 10 out]
  n116 = call "IMAQ Dispose Object Tracking Session"("Object Tracking Session"=w27) -> ()  [unwired: 1 in, 10 out]
  n117 = call "IMAQ Dispose Object Tracking Session"("Object Tracking Session"=w49) -> ()  [unwired: 1 in, 10 out]
  n118 = call <vilib>:"IMAQdx Close Camera.vi"("Session In"=w26) -> ()  [unwired: 10 in, 1 out]
  n119 = call <vilib>:"IMAQdx Close Camera.vi"("Session In"=w69) -> ()  [unwired: 10 in, 1 out]
